vi "Construct Configuration Object.vi"(6 "Group Name":string, 7 "Window Title":string, 8 "error in (no error)":errorcluster, 9 "Initial Category Selection":i32=-1, 10 "Configuration File Path":path, 11 "Configuration in":refnum<class "Configuration.lvclass">) -> (0 "error out":errorcluster, 1 "Stop Event":refnum<user-event>, 2 "Path to config file":path, 3 "Configuration out":refnum<class "Configuration.lvclass">)   [LabVIEW 2026, in "Configuration.lvlib" / "Configuration.lvclass"]
uses:
  Configuration.lvclass
  <vilib>/Utility/sysdir.llb/System Directory Type.ctl
  Configuration.lvclass/Configuration.ctl
  recovery/packages/oglib_file-4.0.1.22-8A89CE420A/File Group 0/user.lib/_OpenG.lib/file/file.llb/Valid Path - Traditional__ogtk.vi
  recovery/packages/oglib_file-4.0.1.22-8A89CE420A/File Group 0/user.lib/_OpenG.lib/file/file.llb/File Exists - Scalar__ogtk.vi
  recovery/packages/oglib_file-4.0.1.22-8A89CE420A/File Group 0/user.lib/_OpenG.lib/file/file.llb/Convert File Extension (Path)__ogtk.vi
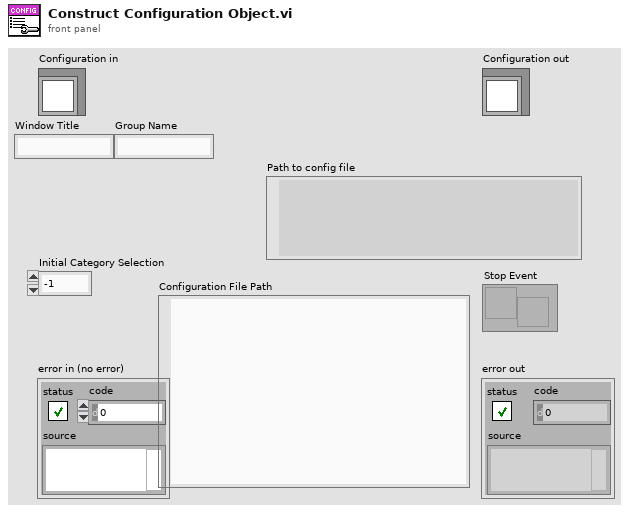
[diagram p1: front panel]
types:
  T1 = typedef "System Directory Type.ctl" = i32
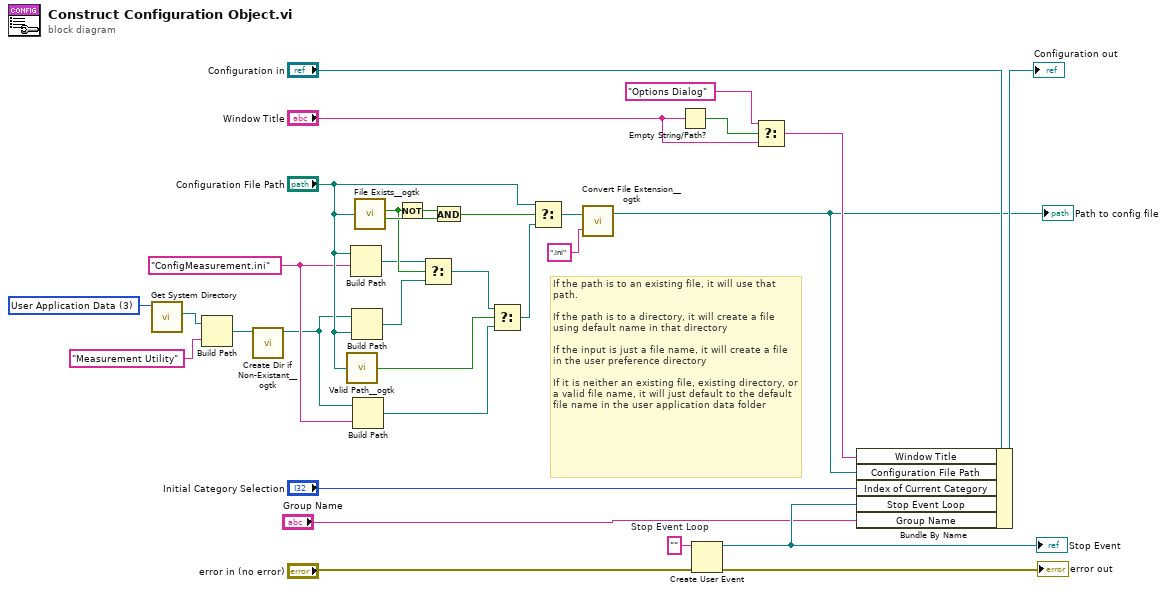
[diagram p0: block diagram]
diagram:
  w13 = "ConfigMeasurement.ini" ("name or relative path")
  w22 = T1 3 items=["User Home"=0, "User Desktop"=1, "User Documents"=2, "User Application Data"=3, "User Preferences"=4, "User Temporary"=5, "Public Documents"=6, "Public Application Data"=7, "Public Preferences"=8, "Public Cache"=13, "System Core Libraries"=9, "System Installed Libraries"=10, "Application Files"=11, "Boot Volume Root"=12] ("system directory type")
  w29 = ""  # Stop Event Loop
  # "If the path is to an existing file, it will use that path.\n\nIf the path is to a directory, it will create a file using default name in that directory\n\nIf the input is just a file name, it will create a file in the user preference directory\n\nIf it is neither an existing file, existing directory, or a valid file name, it will just default to the default file name in the user application data folder"
  n1 = call <vilib>:"Get System Directory.vi"("system directory type"=w22) -> ("system directory"=w5:path)  [unwired: 10 in]
  n2 = Build Path(base path=w5, name or relative path="Measurement Utility") -> (appended path=w3:path)
  n3 = call "Create Dir if Non-Existant__ogtk.vi"("Directory Path"=w3) -> ("dup Directory Path"=w2:path)  [unwired: 8 in, 2 out]
  n4 = call-poly "Valid Path__ogtk.vi"("path"="Configuration File Path") -> ("valid"=w12:bool)
  n5 = Build Path(base path="Configuration File Path", name or relative path=w13) -> (appended path=w16:path)
  n6 = Build Path(base path=w2, name or relative path="Configuration File Path") -> (appended path=w15:path)
  n7 = Build Path(base path=w2, name or relative path=w13) -> (appended path=w11:path)
  n8 = call-poly "File Exists__ogtk.vi"("file path"="Configuration File Path") -> ("is directory"=w17:bool, "exists"=w19:bool)  [unwired: 6 in]
  n9 = Not(x=w17) -> (.not. x?=w20:bool)
  n10 = Select(t=w16, s=w17, f=w15) -> (s? t:f=w10:path)
  n11 = And(x=w20, y=w19) -> (x .and. y?=w18:bool)
  n12 = Select(t=w10, s=w12, f=w11) -> (s? t:f=w9:path)
  n13 = Select(t="Configuration File Path", s=w18, f=w9) -> (s? t:f=w8:path)
  n14 = call-poly "Convert File Extension__ogtk.vi"("new ending (none)"=".ini" ("y"), "file name"=w8) -> ("new filename"=w6:path)  [unwired: 1 out]
  "Path to config file" <- w6
  n15 = Empty String/Path?(string/path="Window Title") -> (empty?=w26:bool)
  n16 = Create User Event(user event datatype=w29, error in="error in (no error)") -> (user event=w30:refnum<user-event>, error out=→"error out":errorcluster)
  "Stop Event" <- w30
  n17 = Select(t="Options Dialog" ("Window Title"), s=w26, f="Window Title") -> (s? t:f=w23:string)
  n18 = Bundle By Name(cluster="Configuration in", "Window Title"=w23, "Configuration File Path"=w6, "Index of Current Category"="Initial Category Selection", "Stop Event Loop"=w30, "Group Name"="Group Name") -> (→"Configuration out":refnum<class "Configuration.lvclass">)
